vi "ATT M2X API.vi"(6 "Food Temp":dbl, 7 "Sunshine":dbl, 8 "elevation":dbl, 9 "longitude":dbl, 10 "latitude":dbl, 11 "M2X Action":T1) -> ()   [LabVIEW 2013]
uses:
  Controls/ATT M2X Streams.ctl
  <vilib>/httpClient/POSTBuffer.vi
  <vilib>/httpClient/PUTBuffer.vi
  <vilib>/httpClient/LabVIEWHTTPClient.lvlib
panel:
  out "JSON string":string
  out "URL":string
  out "Response Body":string
  out "Headers":string
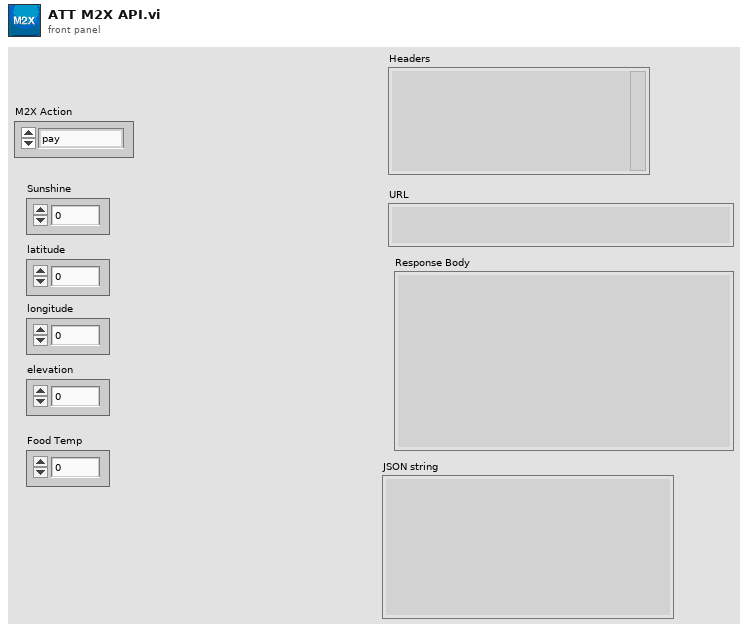
[diagram p1: front panel]
types:
  T1 = typedef "ATT M2X Streams.ctl" = enum16{"pay", "deliver", "sunshine", "location", "temp"}
  T2 = typedef "LabVIEWHTTPClient.lvlib/ClientHandle.ctl" = refnum<k1>
  T3 = cluster{"name":string, "elevation":dbl, "latitude":dbl, "longitude":dbl}
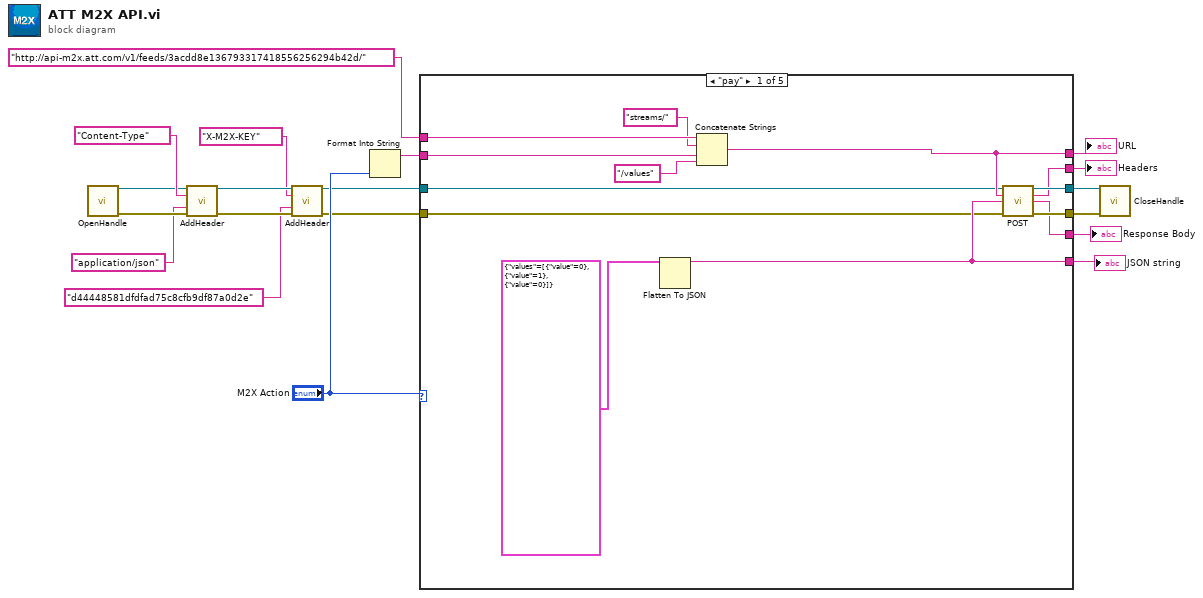
[diagram p0: block diagram]
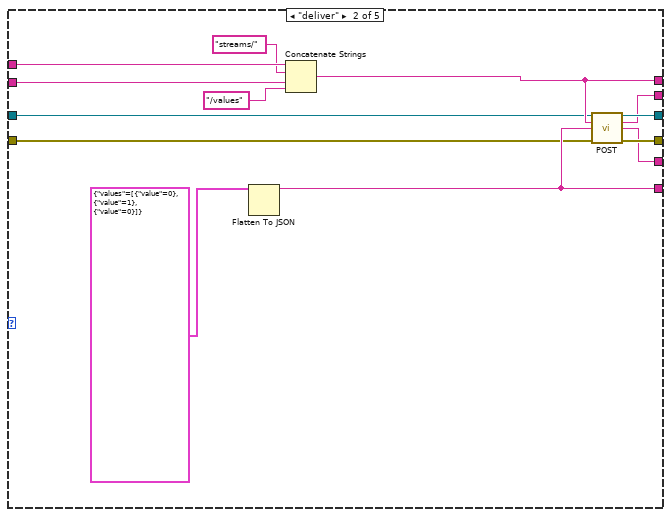
[diagram p2: hidden frame]
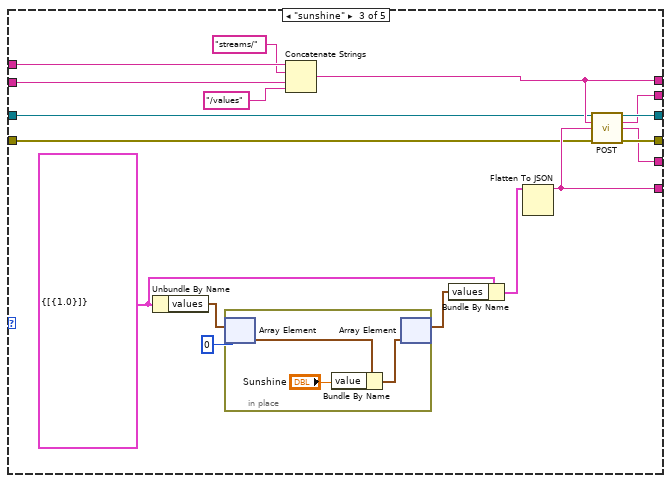
[diagram p3: hidden frame]
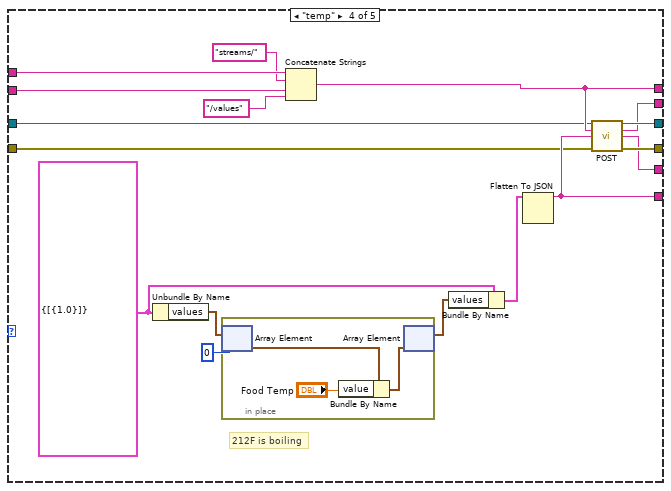
[diagram p4: hidden frame]
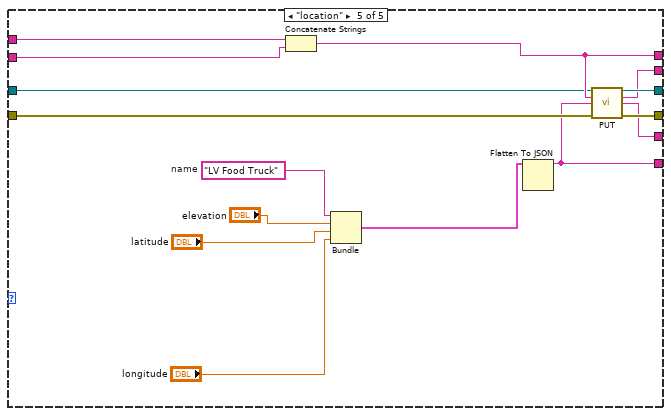
[diagram p5: hidden frame]
diagram:
  n1 = call <vilib>:"OpenHandle.vi"() -> ("client handle out"=w15:T2, "error out"=w18:errorcluster)  [unwired: 14 in]
  n2 = call <vilib>:"AddHeader.vi"("client handle"=w15, "header"="Content-Type", "value"="application/json", "error in (no error)"=w18) -> ("client handle out"=w14:T2, "error out"=w13:errorcluster)  [unwired: 10 in]
  n3 = call <vilib>:"AddHeader.vi"("client handle"=w14, "header"="X-M2X-KEY", "value"="d44448581dfdfad75c8cfb9df87a0d2e", "error in (no error)"=w13) -> ("client handle out"=w10:T2, "error out"=w9:errorcluster)  [unwired: 10 in]
  n4 = Format Into String("M2X Action") -> (resulting string=w8:string)  [unwired: 3 in, 1 out]
  n5 = case shown="\"pay\"" "M2X Action" {
    tunnel: [w22 w35 w53 w73 w93] -> w1
    tunnel: w10 -> [w20 w33 w51 w71 w92]
    tunnel: [w27 w40 w58 w78 w98] -> w5
    tunnel: w9 -> [w21 w34 w52 w72 w100]
    tunnel: [w26 w39 w57 w77 w97] -> w6
    tunnel: [w23 w36 w54 w74 w94] -> w2
    tunnel: w8 -> [w28 w41 w59 w79 w86]
    tunnel: "http://api-m2x.att.com/v1/feeds/3acdd8e136793317418556256294b42d/" ("url") -> [w30 w43 w61 w81 w99]
    tunnel: [w25 w38 w56 w76 w96] -> w4
    tunnel: [w24 w37 w55 w75 w95] -> w3
    frame "pay" {
      n6 = Flatten To JSON(anything=cluster{"values":cluster{"value":i32}[]} {"values"=[{"value"=0}, {"value"=1}, {"value"=0}]}) -> (JSON string=w22:string)  [unwired: 2 in, 1 out]
      n7 = Concatenate Strings(w30, "streams/" ("string"), w28, "/values" ("string")) -> (w23:string)
      n8 = call-poly <vilib>:"POST.vi"("client handle"=w20, "url"=w23, "buffer"=w22, "error in (no error)"=w21) -> ("client handle out"=w27:T2, "headers"=w25:string, "body"=w24:string, "error out"=w26:errorcluster)  [unwired: 8 in]
    }
    frame "deliver" {
      n9 = Flatten To JSON(anything=cluster{"values":cluster{"value":i32}[]} {"values"=[{"value"=0}, {"value"=1}, {"value"=0}]}) -> (JSON string=w35:string)  [unwired: 2 in, 1 out]
      n10 = Concatenate Strings(w43, "streams/" ("string"), w41, "/values" ("string")) -> (w36:string)
      n11 = call-poly <vilib>:"POST.vi"("client handle"=w33, "url"=w36, "buffer"=w35, "error in (no error)"=w34) -> ("client handle out"=w40:T2, "headers"=w38:string, "body"=w37:string, "error out"=w39:errorcluster)  [unwired: 8 in]
    }
    frame "sunshine" {
      w48 = cluster{"values":cluster{"value":dbl}[]} {"values"=[{"value"=1.0}]}
      n12 = Unbundle By Name(w48) -> ("values"=w50:cluster{"value":dbl}[])
      n13 = in-place {
        n14 = in-place-array #1(w50, 0) -> (w64:cluster{"value":dbl})
        n15 = Bundle By Name(cluster=w64, "value"="Sunshine") -> (w63:cluster{"value":dbl})
        n16 = in-place-array #1(w63) -> (w47:cluster{"value":dbl}[])  [unwired: 1 out]
      }
      n17 = Concatenate Strings(w61, "streams/" ("string"), w59, "/values" ("string")) -> (w54:string)
      n18 = Bundle By Name(cluster=w48, "values"=w47) -> (w46:cluster{"values":cluster{"value":dbl}[]})
      n19 = Flatten To JSON(anything=w46) -> (JSON string=w53:string)  [unwired: 2 in, 1 out]
      n20 = call-poly <vilib>:"POST.vi"("client handle"=w51, "url"=w54, "buffer"=w53, "error in (no error)"=w52) -> ("client handle out"=w58:T2, "headers"=w56:string, "body"=w55:string, "error out"=w57:errorcluster)  [unwired: 8 in]
    }
    frame "temp" {
      w68 = cluster{"values":cluster{"value":dbl}[]} {"values"=[{"value"=1.0}]}
      # "212F is boiling"
      n21 = Unbundle By Name(w68) -> ("values"=w70:cluster{"value":dbl}[])
      n22 = in-place {
        n23 = in-place-array #2(w70, 0) -> (w84:cluster{"value":dbl})
        n24 = Bundle By Name(cluster=w84, "value"="Food Temp") -> (w83:cluster{"value":dbl})
        n25 = in-place-array #2(w83) -> (w67:cluster{"value":dbl}[])  [unwired: 1 out]
      }
      n26 = Concatenate Strings(w81, "streams/" ("string"), w79, "/values" ("string")) -> (w74:string)
      n27 = Bundle By Name(cluster=w68, "values"=w67) -> (w66:cluster{"values":cluster{"value":dbl}[]})
      n28 = Flatten To JSON(anything=w66) -> (JSON string=w73:string)  [unwired: 2 in, 1 out]
      n29 = call-poly <vilib>:"POST.vi"("client handle"=w71, "url"=w74, "buffer"=w73, "error in (no error)"=w72) -> ("client handle out"=w78:T2, "headers"=w76:string, "body"=w75:string, "error out"=w77:errorcluster)  [unwired: 8 in]
    }
    frame "location" {
      w91 = "LV Food Truck"  # name
      n30 = Concatenate Strings(w99, w86) -> (w94:string)
      n31 = Bundle("name"=w91, "elevation"="elevation", "latitude"="latitude", "longitude"="longitude") -> (w87:T3)  [unwired: 1 in]
      n32 = Flatten To JSON(anything=w87) -> (JSON string=w93:string)  [unwired: 2 in, 1 out]
      n33 = call-poly <vilib>:"PUT.vi"("client handle"=w92, "url"=w94, "buffer"=w93, "error in (no error)"=w100) -> ("client handle out"=w98:T2, "headers"=w96:string, "body"=w95:string, "error out"=w97:errorcluster)  [unwired: 8 in]
    }
  }
  "Headers" <- w4
  "Response Body" <- w3
  "URL" <- w2
  "JSON string" <- w1
  n34 = call <vilib>:"CloseHandle.vi"("client handle"=w5, "error in (no error)"=w6) -> ()  [unwired: 13 in, 1 out]
